vi "Headless Modular Test.vi"(11 "Path":path) -> ()   [LabVIEW 2018]
uses:
  Classes/Message/Message.lvclass
  49767ad8-b7f6-4460-8d0b-c214da006980.vi
  Classes/STOP Message/STOP.lvclass
  C:/Users/aaron.jencks/Documents/GitHub/emerson_seed_object_detection/LabVIEW/Projects/Paul's Video Viewer/Classes/Message/Message.lvclass
  Classes/Frame Data Message/Frame Data Message.lvclass
  Classes/Video Processor/Video Processor.lvclass
  Classes/Headless Image Processing Handler/Headless Image Processing Handler.lvclass
panel:
  out "Progress":dbl(slide) scale=0.0..100.0
  in  "stop":bool
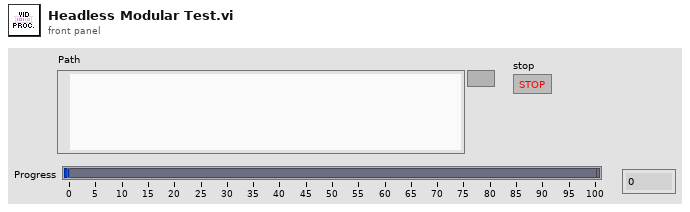
[diagram p1: front panel]
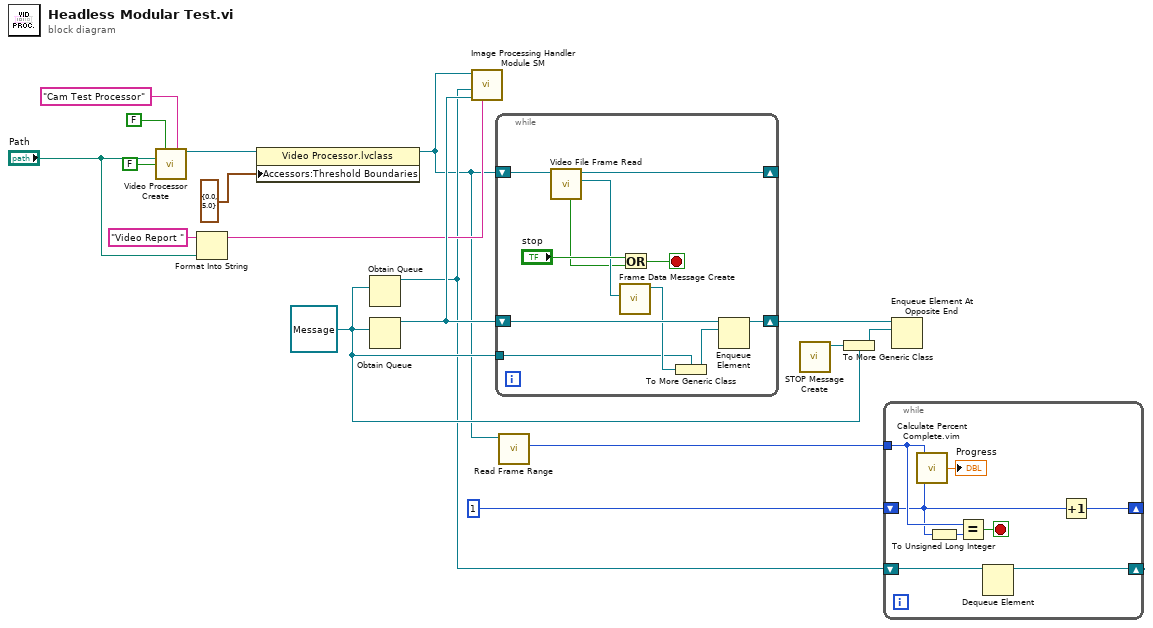
[diagram p0: block diagram]
diagram:
  w8 = refnum<class "Message.lvclass"> refnum ("Message.lvclass")
  n1 = call "Video Processor Create.vi"("Loop? (T)"=FALSE ("Open? (T)"), "Identifier"="Cam Test Processor", "Video Path (\"\")"="Path", "Full? (T)"=FALSE) -> ("Video Processor out"=w11:refnum<class "Video Processor.lvclass">)  [unwired: 10 in, 1 out]
  n2 = Format Into String(initial string="Video Report ", "Path") -> (resulting string=w5:string)  [unwired: 2 in, 1 out]
  n3 = property class="Video Processor.lvclass"(reference=w11, "Accessors:Threshold Boundaries"=cluster{"Minimum":dbl, "Maximum":dbl} {"Minimum"=0.0, "Maximum"=5.0} ("Threshold Boundaries")) -> (reference out=w2:refnum<class "Video Processor.lvclass">)  [unwired: 1 in, 1 out]
  n4 = Obtain Queue(element data type=w8) -> (queue out=w4:refnum<queue>)  [unwired: 4 in, 2 out]
  n5 = Obtain Queue(element data type=w8) -> (queue out=w9:refnum<queue>)  [unwired: 4 in, 2 out]
  n6 = call "Image Processing Handler Module SM.vi"("Identifier"=w5, "data queue"=w9, "tx data queue"=w4, "Video Processor"=w2) -> ()  [unwired: 8 in]
  n7 = while {
    shift-right: [w18] -> _
    shift-left: w2 -> [w28]
    tunnel: w8 -> [w23]
    shift-right: [w21] -> w17
    shift-left: w9 -> [w25]
    stop <- w20 stop-if-true
    n8 = call-dynamic "Video File Frame Read.vi"("Video Processor in"=w28) -> ("Video Frame out"=w26:refnum<class "Video Frame.lvclass">, "Video Processor out"=w18:refnum<class "Video Processor.lvclass">, "Playback Finished?"=w19:bool)  [unwired: 6 in, 2 out]
    n9 = call "Frame Data Message Create.vi"("Video Frame"=w26) -> ("Frame Data Message out"=w24:refnum<class "Frame Data Message.lvclass">)  [unwired: 9 in, 1 out]
    n10 = Or(x="stop", y=w19) -> (x .or. y?=w20:bool)
    n11 = To More Generic Class(target class=w23, reference=w24) -> (generic class reference=w22:refnum<class "Message.lvclass">)
    n12 = Enqueue Element(queue=w25, element=w22) -> (queue out=w21:refnum<queue>)  [unwired: 2 in, 2 out]
  }
  n13 = call-dynamic "Read Frame Range.vi"("Video File in"=w2) -> ("Number of Frames"=w1:u32)  [unwired: 8 in, 2 out]
  n14 = call "STOP Message Create.vi"() -> ("STOP out"=w16:refnum<class "STOP.lvclass">)  [unwired: 10 in, 1 out]
  n15 = To More Generic Class(target class=w8, reference=w16) -> (generic class reference=w15:refnum<class "Message.lvclass">)
  n16 = while {
    shift-right: [w35] -> _
    shift-left: w4 -> [w36]
    shift-right: [w34] -> _
    shift-left: 1 -> [w31]
    tunnel: w1 -> [w32]
    stop <- w30 stop-if-true
    n17 = call "Calculate Percent Complete.vim"("Total"=w31, "Part"=w32) -> ("% Complete"=→"Progress":dbl)
    n18 = To Unsigned Long Integer(number=w31) -> (unsigned 32bit integer=w29:u32)
    n19 = Equal?(x=w32, y=w29) -> (x = y?=w30:bool)
    n20 = Dequeue Element(queue=w36) -> (queue out=w35:refnum<queue>)  [unwired: 2 in, 3 out]
    n21 = Increment(x=w31) -> (x+1=w34:i32)
  }
  n22 = Enqueue Element At Opposite End(queue=w17, element=w15) -> ()  [unwired: 2 in, 3 out]
